vi "传感器特性判定.vi"(7 "Result":refnum<vi>, 10 "判定参数":T1, 11 "XY曲线":cluster{"X":dbl[], "Y":dbl[]}[](array[cluster])) -> (2 "判定项长度":i32, 3 "OK？":bool)   [LabVIEW 2019]
uses:
  <vilib>/Analysis/6fits.llb/Curve Fitting Criteria.ctl
  <vilib>/Analysis/NI_AALPro.lvlib
  <vilib>/Analysis/NI_AAL_Geometry.lvlib
panel:
  out "定点设置":dbl
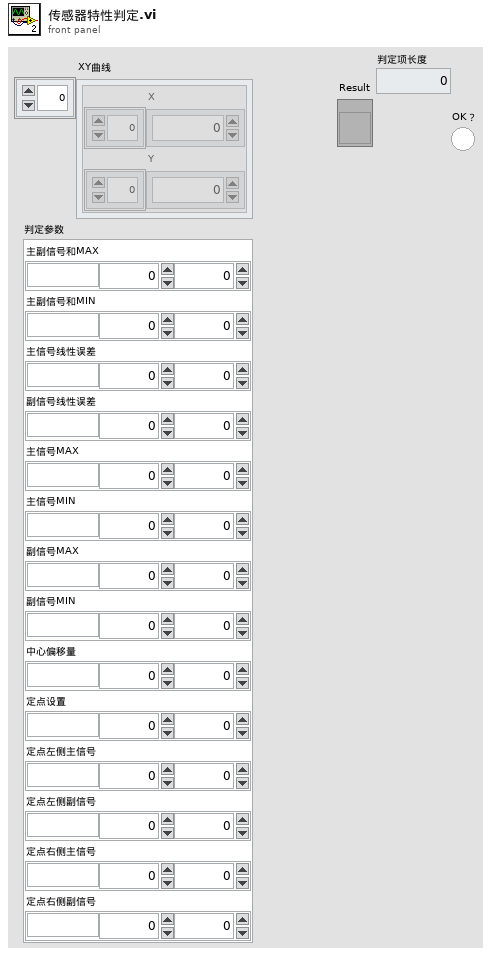
[diagram p1: front panel]
types:
  T1 = cluster{"主副信号和MAX":cluster{"单位":string, "下限":dbl, "上限":dbl}, "主副信号和MIN":cluster{"单位":string, "下限":dbl, "上限":dbl}, "主信号线性误差":cluster{"单位":string, "下限":dbl, "上限":dbl}, "副信号线性误差":cluster{"单位":string, "下限":dbl, "上限":dbl}, "主信号MAX":cluster{"单位":string, "下限":dbl, "上限":dbl}, "主信号MIN":cluster{"单位":string, "下限":dbl, "上限":dbl}, "副信号MAX":cluster{"单位":string, "下限":dbl, "上限":dbl}, "副信号MIN":cluster{"单位":string, "下限":dbl, "上限":dbl}, "中心偏移量":cluster{"单位":string, "下限":dbl, "上限":dbl}, "定点设置":cluster{"单位":string, "下限":dbl, "上限":dbl}, "定点左侧主信号":cluster{"单位":string, "下限":dbl, "上限":dbl}, "定点左侧副信号":cluster{"单位":string, "下限":dbl, "上限":dbl}, "定点右侧主信号":cluster{"单位":string, "下限":dbl, "上限":dbl}, "定点右侧副信号":cluster{"单位":string, "下限":dbl, "上限":dbl}}
  T2 = typedef "NI_AALPro.lvlib/Curve Fitting Criteria.ctl" = u16
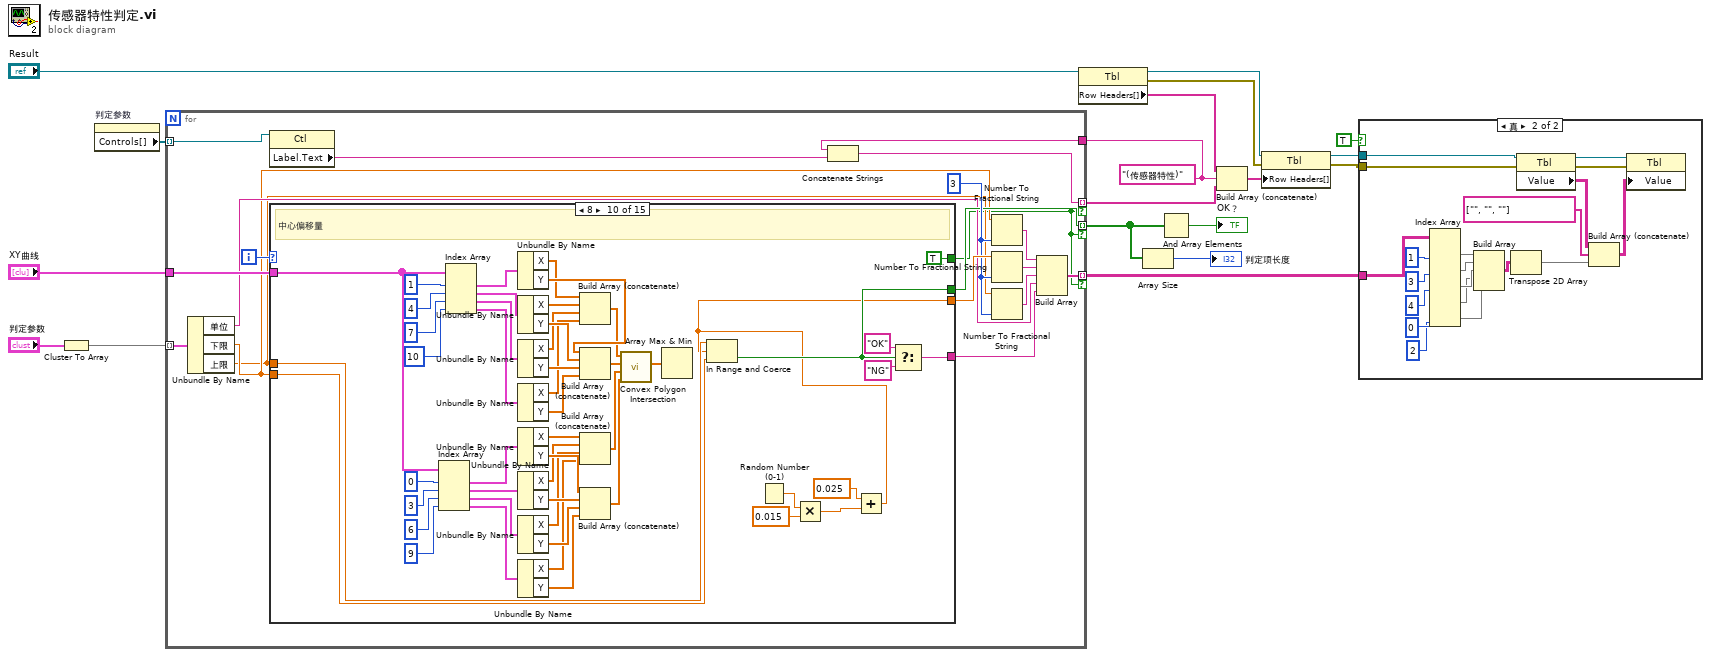
[diagram p0: block diagram]
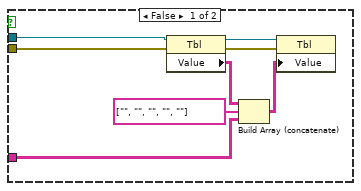
[diagram p2: hidden frame]
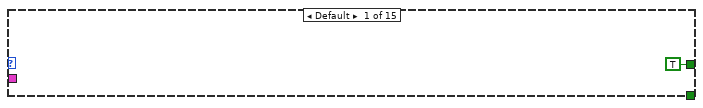
[diagram p3: hidden frame]
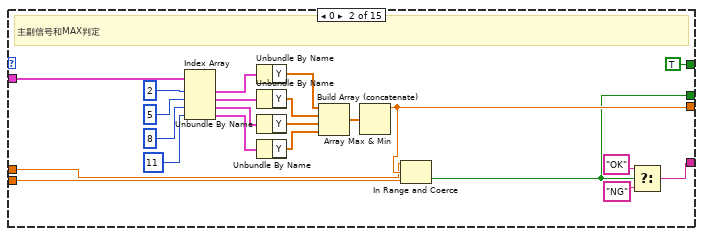
[diagram p4: hidden frame]
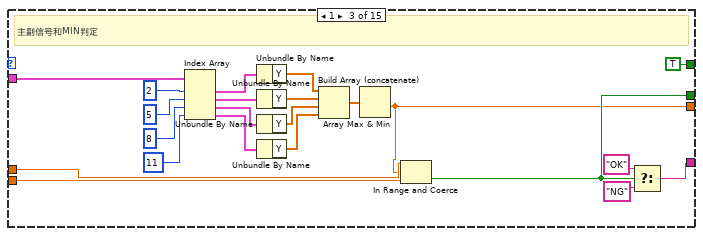
[diagram p5: hidden frame]
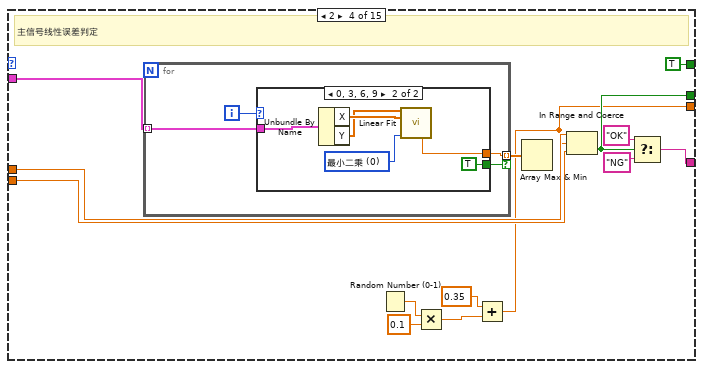
[diagram p6: hidden frame]
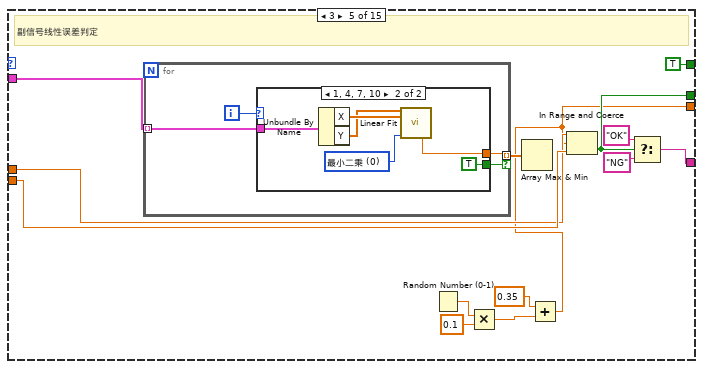
[diagram p8: hidden frame]
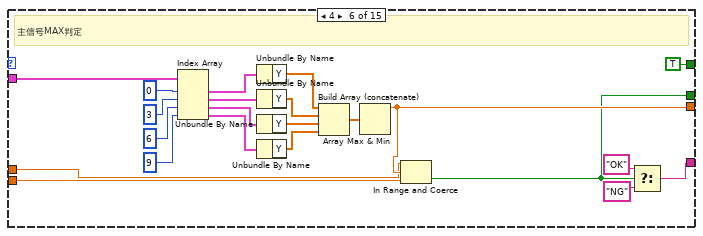
[diagram p10: hidden frame]
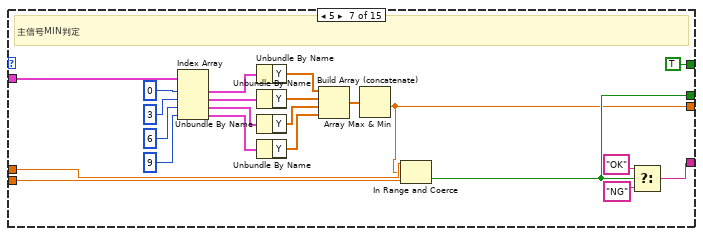
[diagram p11: hidden frame]
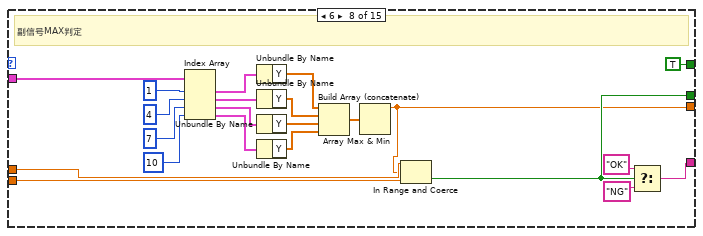
[diagram p12: hidden frame]
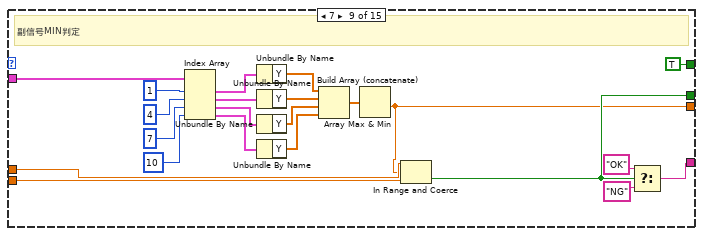
[diagram p13: hidden frame]
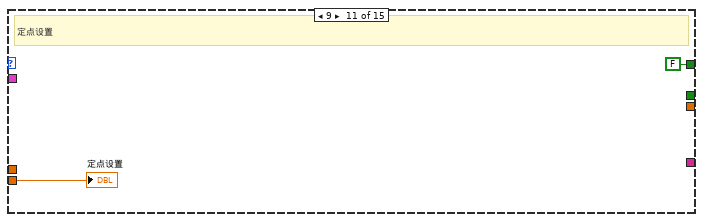
[diagram p14: hidden frame]
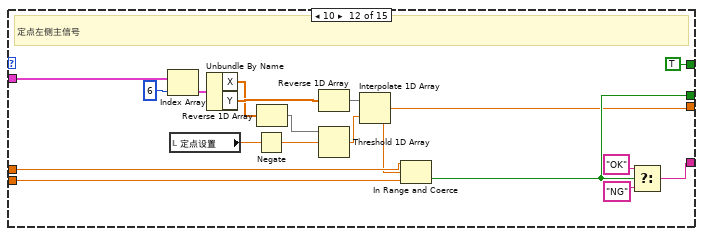
[diagram p15: hidden frame]
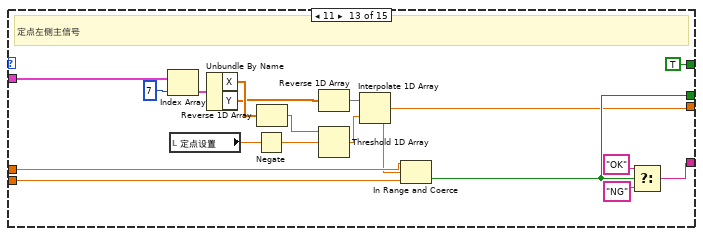
[diagram p16: hidden frame]
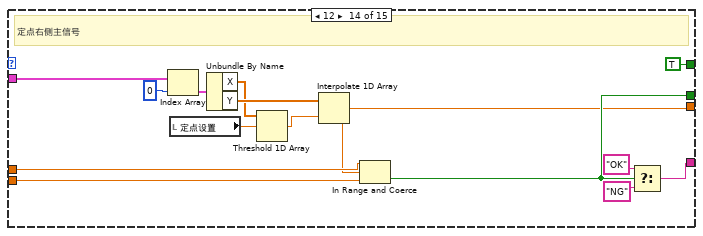
[diagram p17: hidden frame]
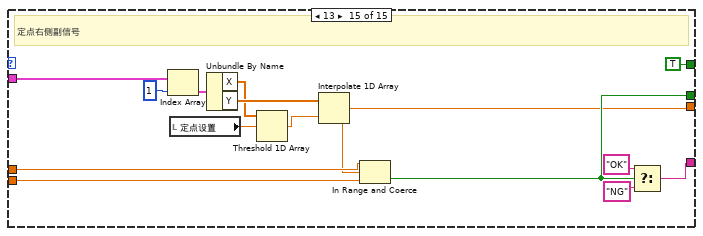
[diagram p18: hidden frame]
diagram:
  w1 = "(传感器特性)" ("Label.Text")
  n1 = Cluster To Array(cluster="判定参数") -> (array=w18:cluster{"单位":string, "下限":dbl, "上限":dbl}[])
  n2 = property on="判定参数" class="Clust (严格)"() -> ("Controls[]"=w16:refnum<vi>[])  [unwired: 2 in, 2 out]
  n3 = for {
    tunnel: w18 -> [w37] mode=indexing
    tunnel: w16 -> [w35] mode=indexing
    tunnel: "XY曲线" -> [w33]
    tunnel: [w27] -> w3 mode=indexing if=w21
    tunnel: [w23] -> w5 mode=indexing if=w21
    tunnel: [w20] -> w8 mode=indexing if=w21
    tunnel: w1 -> [w19]
    i -> [w36]
    w32 = i16 3 ("精度(6)")
    n4 = Unbundle By Name(w37) -> ("单位"=w26:string, "下限"=w25:dbl, "上限"=w24:dbl)
    n5 = property class="Ctl"(reference=w35) -> ("Label.Text"=w22:string)  [unwired: 1 in, 2 out]
    n6 = case shown="8" w36 {
      tunnel: [_ w46 w61 w83 w107 w138 w154 w176 w198 w219 _ w275 w292 w309 w324] -> w34
      tunnel: w33 -> [_ w60 w82 w89 w113 w152 w174 w196 w218 w237 _ w288 w306 w321 w336]
      tunnel: [_ w43 w66 w94 w118 w135 w158 w180 w202 w254 _ w284 w302 w317 w332] -> w28
      tunnel: [_ w42 w65 w93 w117 w134 w157 w179 w201 w253 _ w283 w301 w316 w331] -> w27
      tunnel: w25 -> [_ w41 w64 w92 w116 w133 w156 w178 w200 w252 w269 w282 w300 w315 w330]
      tunnel: w24 -> [_ w40 w63 w91 w115 w132 w155 w177 w199 w251 _ w281 w299 w314 w329]
      tunnel: [TRUE TRUE TRUE TRUE TRUE TRUE TRUE TRUE TRUE TRUE FALSE TRUE TRUE TRUE TRUE] -> w21
      frame Default {
      }
      frame 0 {
        # "主副信号和MAX判定"
        n7 = Index Array(array=w60, index #1=2 ("索引"), index #2=5 ("索引"), index #3=8 ("索引"), index #4=11 ("索引")) -> (element #1=w55:cluster{"X":dbl[], "Y":dbl[]}, element #2=w52:cluster{"X":dbl[], "Y":dbl[]}, element #3=w53:cluster{"X":dbl[], "Y":dbl[]}, element #4=w54:cluster{"X":dbl[], "Y":dbl[]})
        n8 = Unbundle By Name(w55) -> ("Y"=w51:dbl[])
        n9 = Unbundle By Name(w52) -> ("Y"=w50:dbl[])
        n10 = Unbundle By Name(w53) -> ("Y"=w49:dbl[])
        n11 = Unbundle By Name(w54) -> ("Y"=w48:dbl[])
        n12 = Build Array (concatenate)(w51, w50, w49, w48) -> (w47:dbl[])
        n13 = Array Max & Min(array=w47) -> (max value=w46:dbl)  [unwired: 3 out]
        n14 = In Range and Coerce(upper limit=w40, x=w46, lower limit=w41) -> (In Range?=w42:bool)  [unwired: 1 out]
        n15 = Select(t="OK", s=w42, f="NG") -> (s? t:f=w43:string)
      }
      frame 1 {
        # "主副信号和MIN判定"
        n16 = Index Array(array=w82, index #1=2 ("索引"), index #2=5 ("索引"), index #3=8 ("索引"), index #4=11 ("索引")) -> (element #1=w77:cluster{"X":dbl[], "Y":dbl[]}, element #2=w74:cluster{"X":dbl[], "Y":dbl[]}, element #3=w75:cluster{"X":dbl[], "Y":dbl[]}, element #4=w76:cluster{"X":dbl[], "Y":dbl[]})
        n17 = Unbundle By Name(w77) -> ("Y"=w73:dbl[])
        n18 = Unbundle By Name(w74) -> ("Y"=w72:dbl[])
        n19 = Unbundle By Name(w75) -> ("Y"=w71:dbl[])
        n20 = Unbundle By Name(w76) -> ("Y"=w70:dbl[])
        n21 = Build Array (concatenate)(w73, w72, w71, w70) -> (w69:dbl[])
        n22 = Array Max & Min(array=w69) -> (min value=w61:dbl)  [unwired: 3 out]
        n23 = In Range and Coerce(upper limit=w63, x=w61, lower limit=w64) -> (In Range?=w65:bool)  [unwired: 1 out]
        n24 = Select(t="OK", s=w65, f="NG") -> (s? t:f=w66:string)
      }
      frame 2 {
        # "主信号线性误差判定"
        n25 = for {
          tunnel: w89 -> [w99] mode=indexing
          tunnel: [w98] -> w88 mode=indexing if=w97
          i -> [w100]
          n26 = case shown="0, 3, 6, 9" w100 {
            tunnel: w99 -> [_ w106]
            tunnel: [_ w104] -> w98
            tunnel: [_ TRUE] -> w97
            frame Default {
            }
            frame 0, 3, 6, 9 {
              w105 = T2 0 items=["最小二乘", "最小绝对残差", "Bisquare"] ("method")
              n27 = Unbundle By Name(w106) -> ("X"=w102:dbl[], "Y"=w101:dbl[])
              n28 = call <vilib>:"Linear Fit.vi"("Y"=w101, "X"=w102, "method"=w105) -> ("residue"=w104:dbl)  [unwired: 8 in, 4 out]
            }
          }
        }
        n29 = Random Number (0-1)() -> (number: 0 to 1=w87:dbl)
        n30 = Multiply(x=w87, y=0.1) -> (x*y=w84:dbl)
        n31 = Add(x=0.35 ("y"), y=w84) -> (x+y=w83:dbl)
        n32 = Array Max & Min(array=w88) -> ()  [unwired: 4 out]
        n33 = In Range and Coerce(upper limit=w91, x=w83, lower limit=w92) -> (In Range?=w93:bool)  [unwired: 1 out]
        n34 = Select(t="OK", s=w93, f="NG") -> (s? t:f=w94:string)
      }
      frame 3 {
        # "副信号线性误差判定"
        n35 = for {
          tunnel: w113 -> [w123] mode=indexing
          tunnel: [w122] -> w112 mode=indexing if=w121
          i -> [w124]
          n36 = case shown="1, 4, 7, 10" w124 {
            tunnel: w123 -> [_ w130]
            tunnel: [_ w128] -> w122
            tunnel: [_ TRUE] -> w121
            frame Default {
            }
            frame 1, 4, 7, 10 {
              w129 = T2 0 items=["最小二乘", "最小绝对残差", "Bisquare"] ("method")
              n37 = Unbundle By Name(w130) -> ("X"=w126:dbl[], "Y"=w125:dbl[])
              n38 = call <vilib>:"Linear Fit.vi"("Y"=w125, "X"=w126, "method"=w129) -> ("residue"=w128:dbl)  [unwired: 8 in, 4 out]
            }
          }
        }
        n39 = Random Number (0-1)() -> (number: 0 to 1=w111:dbl)
        n40 = Multiply(x=w111, y=0.1) -> (x*y=w110:dbl)
        n41 = Array Max & Min(array=w112) -> ()  [unwired: 4 out]
        n42 = Add(x=0.35 ("y"), y=w110) -> (x+y=w107:dbl)
        n43 = In Range and Coerce(upper limit=w115, x=w107, lower limit=w116) -> (In Range?=w117:bool)  [unwired: 1 out]
        n44 = Select(t="OK", s=w117, f="NG") -> (s? t:f=w118:string)
      }
      frame 4 {
        # "主信号MAX判定"
        n45 = Index Array(array=w152, index #1=0 ("索引"), index #2=3 ("索引"), index #3=6 ("索引"), index #4=9 ("索引")) -> (element #1=w147:cluster{"X":dbl[], "Y":dbl[]}, element #2=w144:cluster{"X":dbl[], "Y":dbl[]}, element #3=w145:cluster{"X":dbl[], "Y":dbl[]}, element #4=w146:cluster{"X":dbl[], "Y":dbl[]})
        n46 = Unbundle By Name(w147) -> ("Y"=w143:dbl[])
        n47 = Unbundle By Name(w144) -> ("Y"=w142:dbl[])
        n48 = Unbundle By Name(w145) -> ("Y"=w141:dbl[])
        n49 = Unbundle By Name(w146) -> ("Y"=w140:dbl[])
        n50 = Build Array (concatenate)(w143, w142, w141, w140) -> (w139:dbl[])
        n51 = Array Max & Min(array=w139) -> (max value=w138:dbl)  [unwired: 3 out]
        n52 = In Range and Coerce(upper limit=w132, x=w138, lower limit=w133) -> (In Range?=w134:bool)  [unwired: 1 out]
        n53 = Select(t="OK", s=w134, f="NG") -> (s? t:f=w135:string)
      }
      frame 5 {
        # "主信号MIN判定"
        n54 = Index Array(array=w174, index #1=0 ("索引"), index #2=3 ("索引"), index #3=6 ("索引"), index #4=9 ("索引")) -> (element #1=w169:cluster{"X":dbl[], "Y":dbl[]}, element #2=w166:cluster{"X":dbl[], "Y":dbl[]}, element #3=w167:cluster{"X":dbl[], "Y":dbl[]}, element #4=w168:cluster{"X":dbl[], "Y":dbl[]})
        n55 = Unbundle By Name(w169) -> ("Y"=w165:dbl[])
        n56 = Unbundle By Name(w166) -> ("Y"=w164:dbl[])
        n57 = Unbundle By Name(w167) -> ("Y"=w163:dbl[])
        n58 = Unbundle By Name(w168) -> ("Y"=w162:dbl[])
        n59 = Build Array (concatenate)(w165, w164, w163, w162) -> (w161:dbl[])
        n60 = Array Max & Min(array=w161) -> (min value=w154:dbl)  [unwired: 3 out]
        n61 = In Range and Coerce(upper limit=w155, x=w154, lower limit=w156) -> (In Range?=w157:bool)  [unwired: 1 out]
        n62 = Select(t="OK", s=w157, f="NG") -> (s? t:f=w158:string)
      }
      frame 6 {
        # "副信号MAX判定"
        n63 = Index Array(array=w196, index #1=1 ("索引"), index #2=4 ("索引"), index #3=7 ("索引"), index #4=10 ("索引")) -> (element #1=w191:cluster{"X":dbl[], "Y":dbl[]}, element #2=w188:cluster{"X":dbl[], "Y":dbl[]}, element #3=w189:cluster{"X":dbl[], "Y":dbl[]}, element #4=w190:cluster{"X":dbl[], "Y":dbl[]})
        n64 = Unbundle By Name(w191) -> ("Y"=w187:dbl[])
        n65 = Unbundle By Name(w188) -> ("Y"=w186:dbl[])
        n66 = Unbundle By Name(w189) -> ("Y"=w185:dbl[])
        n67 = Unbundle By Name(w190) -> ("Y"=w184:dbl[])
        n68 = Build Array (concatenate)(w187, w186, w185, w184) -> (w183:dbl[])
        n69 = Array Max & Min(array=w183) -> (max value=w176:dbl)  [unwired: 3 out]
        n70 = In Range and Coerce(upper limit=w177, x=w176, lower limit=w178) -> (In Range?=w179:bool)  [unwired: 1 out]
        n71 = Select(t="OK", s=w179, f="NG") -> (s? t:f=w180:string)
      }
      frame 7 {
        # "副信号MIN判定"
        n72 = Index Array(array=w218, index #1=1 ("索引"), index #2=4 ("索引"), index #3=7 ("索引"), index #4=10 ("索引")) -> (element #1=w213:cluster{"X":dbl[], "Y":dbl[]}, element #2=w210:cluster{"X":dbl[], "Y":dbl[]}, element #3=w211:cluster{"X":dbl[], "Y":dbl[]}, element #4=w212:cluster{"X":dbl[], "Y":dbl[]})
        n73 = Unbundle By Name(w213) -> ("Y"=w209:dbl[])
        n74 = Unbundle By Name(w210) -> ("Y"=w208:dbl[])
        n75 = Unbundle By Name(w211) -> ("Y"=w207:dbl[])
        n76 = Unbundle By Name(w212) -> ("Y"=w206:dbl[])
        n77 = Build Array (concatenate)(w209, w208, w207, w206) -> (w205:dbl[])
        n78 = Array Max & Min(array=w205) -> (min value=w198:dbl)  [unwired: 3 out]
        n79 = In Range and Coerce(upper limit=w199, x=w198, lower limit=w200) -> (In Range?=w201:bool)  [unwired: 1 out]
        n80 = Select(t="OK", s=w201, f="NG") -> (s? t:f=w202:string)
      }
      frame 8 {
        # "中心偏移量"
        n81 = Index Array(array=w237, index #1=0 ("索引"), index #2=3 ("索引"), index #3=6 ("索引"), index #4=9 ("索引")) -> (element #1=w264:cluster{"X":dbl[], "Y":dbl[]}, element #2=w261:cluster{"X":dbl[], "Y":dbl[]}, element #3=w262:cluster{"X":dbl[], "Y":dbl[]}, element #4=w263:cluster{"X":dbl[], "Y":dbl[]})
        n82 = Index Array(array=w237, index #1=1 ("索引"), index #2=4 ("索引"), index #3=7 ("索引"), index #4=10 ("索引")) -> (element #1=w242:cluster{"X":dbl[], "Y":dbl[]}, element #2=w245:cluster{"X":dbl[], "Y":dbl[]}, element #3=w244:cluster{"X":dbl[], "Y":dbl[]}, element #4=w243:cluster{"X":dbl[], "Y":dbl[]})
        n83 = Unbundle By Name(w242) -> ("X"=w236:dbl[], "Y"=w246:dbl[])
        n84 = Unbundle By Name(w245) -> ("X"=w235:dbl[], "Y"=w247:dbl[])
        n85 = Unbundle By Name(w244) -> ("X"=w234:dbl[], "Y"=w248:dbl[])
        n86 = Unbundle By Name(w243) -> ("X"=w233:dbl[], "Y"=w249:dbl[])
        n87 = Unbundle By Name(w264) -> ("X"=w232:dbl[], "Y"=w260:dbl[])
        n88 = Unbundle By Name(w261) -> ("X"=w231:dbl[], "Y"=w259:dbl[])
        n89 = Unbundle By Name(w262) -> ("X"=w230:dbl[], "Y"=w258:dbl[])
        n90 = Unbundle By Name(w263) -> ("X"=w229:dbl[], "Y"=w257:dbl[])
        n91 = Build Array (concatenate)(w236, w235, w234, w233) -> (w226:dbl[])
        n92 = Build Array (concatenate)(w246, w247, w248, w249) -> (w228:dbl[])
        n93 = Build Array (concatenate)(w232, w231, w230, w229) -> (w225:dbl[])
        n94 = Build Array (concatenate)(w260, w259, w258, w257) -> (w224:dbl[])
        n95 = call <vilib>:"Convex Polygon Intersection.vi"("Y 2"=w224, "X 2"=w225, "Y 1"=w228, "X 1"=w226) -> ("Intersection Y"=w227:dbl[])  [unwired: 5 in, 2 out]
        n96 = Array Max & Min(array=w227) -> ()  [unwired: 4 out]
        n97 = Random Number (0-1)() -> (number: 0 to 1=w223:dbl)
        n98 = Multiply(x=w223, y=0.015) -> (x*y=w220:dbl)
        n99 = Add(x=0.025 ("y"), y=w220) -> (x+y=w219:dbl)
        n100 = In Range and Coerce(upper limit=w251, x=w219, lower limit=w252) -> (In Range?=w253:bool)  [unwired: 1 out]
        n101 = Select(t="OK", s=w253, f="NG") -> (s? t:f=w254:string)
      }
      frame 9 {
        # "定点设置"
        "定点设置" <- w269
      }
      frame 10 {
        # "定点左侧主信号"
        n102 = Index Array(array=w288, index=6 ("索引")) -> (element=w287:cluster{"X":dbl[], "Y":dbl[]})
        n103 = local read "定点设置"() -> (w277:dbl)
        n104 = Unbundle By Name(w287) -> ("X"=w274:dbl[], "Y"=w276:dbl[])
        n105 = Negate(x=w277) -> (-x=w273:dbl)
        n106 = Reverse 1D Array(array=w274) -> (reversed array=w272:dbl[])
        n107 = Reverse 1D Array(array=w276) -> (reversed array=w271:dbl[])
        n108 = Threshold 1D Array(2:w273, 3:w272) -> (0:w278:dbl)  [unwired: 1 in]
        n109 = Interpolate 1D Array(1:w278, 2:w271) -> (0:w275:dbl)
        n110 = In Range and Coerce(upper limit=w281, x=w275, lower limit=w282) -> (In Range?=w283:bool)  [unwired: 1 out]
        n111 = Select(t="OK", s=w283, f="NG") -> (s? t:f=w284:string)
      }
      frame 11 {
        # "定点左侧主信号"
        n112 = Index Array(array=w306, index=7 ("索引")) -> (element=w305:cluster{"X":dbl[], "Y":dbl[]})
        n113 = local read "定点设置"() -> (w294:dbl)
        n114 = Unbundle By Name(w305) -> ("X"=w295:dbl[], "Y"=w293:dbl[])
        n115 = Negate(x=w294) -> (-x=w289:dbl)
        n116 = Reverse 1D Array(array=w295) -> (reversed array=w291:dbl[])
        n117 = Reverse 1D Array(array=w293) -> (reversed array=w290:dbl[])
        n118 = Threshold 1D Array(2:w289, 3:w291) -> (0:w296:dbl)  [unwired: 1 in]
        n119 = Interpolate 1D Array(1:w296, 2:w290) -> (0:w292:dbl)
        n120 = In Range and Coerce(upper limit=w299, x=w292, lower limit=w300) -> (In Range?=w301:bool)  [unwired: 1 out]
        n121 = Select(t="OK", s=w301, f="NG") -> (s? t:f=w302:string)
      }
      frame 12 {
        # "定点右侧主信号"
        n122 = Index Array(array=w321, index=0 ("索引")) -> (element=w320:cluster{"X":dbl[], "Y":dbl[]})
        n123 = local read "定点设置"() -> (w307:dbl)
        n124 = Unbundle By Name(w320) -> ("X"=w308:dbl[], "Y"=w310:dbl[])
        n125 = Threshold 1D Array(2:w307, 3:w308) -> (0:w311:dbl)  [unwired: 1 in]
        n126 = Interpolate 1D Array(1:w311, 2:w310) -> (0:w309:dbl)
        n127 = In Range and Coerce(upper limit=w314, x=w309, lower limit=w315) -> (In Range?=w316:bool)  [unwired: 1 out]
        n128 = Select(t="OK", s=w316, f="NG") -> (s? t:f=w317:string)
      }
      frame 13 {
        # "定点右侧副信号"
        n129 = Index Array(array=w336, index=1 ("索引")) -> (element=w335:cluster{"X":dbl[], "Y":dbl[]})
        n130 = local read "定点设置"() -> (w322:dbl)
        n131 = Unbundle By Name(w335) -> ("X"=w323:dbl[], "Y"=w325:dbl[])
        n132 = Threshold 1D Array(2:w322, 3:w323) -> (0:w326:dbl)  [unwired: 1 in]
        n133 = Interpolate 1D Array(1:w326, 2:w325) -> (0:w324:dbl)
        n134 = In Range and Coerce(upper limit=w329, x=w324, lower limit=w330) -> (In Range?=w331:bool)  [unwired: 1 out]
        n135 = Select(t="OK", s=w331, f="NG") -> (s? t:f=w332:string)
      }
    }
    n136 = Concatenate Strings(w19, w22) -> (w20:string)
    n137 = Number To Fractional String(number=w25, precision (6)=w32) -> (F-format string=w31:string)  [unwired: 2 in]
    n138 = Number To Fractional String(number=w34, precision (6)=w32) -> (F-format string=w30:string)  [unwired: 2 in]
    n139 = Number To Fractional String(number=w24, precision (6)=w32) -> (F-format string=w29:string)  [unwired: 2 in]
    n140 = Build Array(w31, w30, w29, w26, w28) -> (w23:string[])
  }
  n141 = property class="Tbl"(reference="Result") -> (reference out=w10:refnum<vi>, error out=w13:errorcluster, "Row Headers[]"=w6:string[])  [unwired: 1 in]
  n142 = Array Size(array=w3) -> (size(s)=→"判定项长度":i32)
  n143 = And Array Elements(Boolean array=w3) -> (logical AND=→"OK？":bool)
  n144 = Build Array (concatenate)(w6, w1, w8) -> (w9:string[])
  n145 = property class="Tbl"(reference=w10, error in=w13, "Row Headers[]"=w9) -> (reference out=w11:refnum<vi>, error out=w12:errorcluster)
  n146 = case shown="真" TRUE {
    tunnel: w12 -> [w342 w362]
    tunnel: w11 -> [w339 w359]
    tunnel: w5 -> [w338 w350]
    frame False {
      n147 = property class="Tbl"(reference=w339, error in=w342) -> (reference out=w340:refnum<vi>, error out=w341:errorcluster, "Value"=w343:string[][])
      n148 = Build Array (concatenate)(w343, string[] ["", "", "", "", ""], w338) -> (w344:string[][])
      n149 = property class="Tbl"(reference=w340, error in=w341, "Value"=w344) -> ()  [unwired: 2 out]
    }
    frame True {
      n150 = Index Array(array=w350, index (col) #1=1 ("禁用的索引 (列)"), index (col) #2=3 ("索引 (列)"), index (col) #3=4 ("索引 (列)"), index (col) #4=0 ("索引 (列)"), index (col) #5=2 ("索引 (列)")) -> (element #1=w354:string[], element #2=w353:string[], element #3=w352:string[], element #4=w346:string[], element #5=w345:string[])  [unwired: 5 in]
      n151 = Build Array(w354, w353, w352, w346, w345) -> (w351:string[][])
      n152 = Transpose 2D Array(2D array=w351) -> (transposed array=w349:string[][])
      n153 = property class="Tbl"(reference=w359, error in=w362) -> (reference out=w360:refnum<vi>, error out=w361:errorcluster, "Value"=w363:string[][])
      n154 = Build Array (concatenate)(w363, string[] ["", "", ""], w349) -> (w364:string[][])
      n155 = property class="Tbl"(reference=w360, error in=w361, "Value"=w364) -> ()  [unwired: 2 out]
    }
  }
